vi "2L04_%-ds-Interv_centre_de_moy_de_lg_n_sigma.vi"(0 "xi":dbl[](array[numeric]), 1 "ni":i16[](array[numeric]), 2 "n":i16, 3 "Moyenne":dbl, 4 "Sigma":dbl) -> (7 "% de +/- n.sigma":dbl, 8 "i deb":i32, 9 "i fin":i32)   [LabVIEW 2010, in "lv_02.lvlib"]
doc: "Dans une distribution gaussienne LN(moyenne, sigma), on cherche dans une distribution expérimentale (xi,ni) le % de l'effectif dans un intervalle centré sur la moyenne à +/- n.sigma.\nSi la moyenne et sigma sont nuls alors, on calculera la moyenne et l'écart-type à partir de la distribution expérimentale."
uses:
  lv_02.lvlib
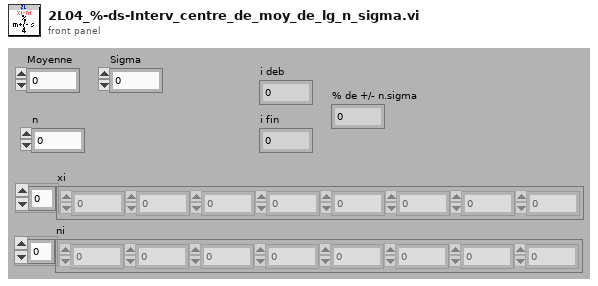
[diagram p1: front panel]
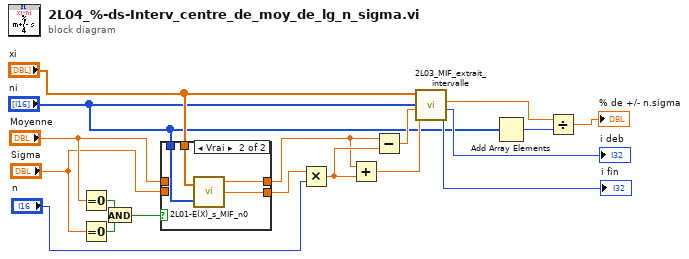
[diagram p0: block diagram]
diagram:
  n1 = Equal To 0?(x="Moyenne") -> (x = 0?=w9:bool)
  n2 = Equal To 0?(x="Sigma") -> (x = 0?=w8:bool)
  n3 = And(x=w9, y=w8) -> (x .and. y?=w7:bool)
  n4 = case shown="Vrai" w7 {
    tunnel: "xi" -> [_ w24]
    tunnel: "ni" -> [_ w23]
    tunnel: [w20 w22] -> w2
    tunnel: [w19 w21] -> w1
    tunnel: "Moyenne" -> [w20 _]
    tunnel: "Sigma" -> [w19 _]
    frame False {
    }
    frame True {
      n5 = call "2L01-E(X)_s_MIF_n0.vi"("ni"=w23, "xic"=w24) -> ("s"=w21:dbl, "E(X)"=w22:dbl)  [unwired: 1 out]
    }
  }
  n6 = Multiply(x=w1, y="n") -> (x*y=w18:dbl)
  n7 = Add(x=w2, y=w18) -> (x+y=w15:dbl)
  n8 = Subtract(x=w2, y=w18) -> (x-y=w16:dbl)
  n9 = call "2L03_MIF_extrait_intervalle.vi"("X fin"=w15, "X deb"=w16, "N"="ni", "X"="xi") -> ("i fin"=→"i fin":i32, "i deb"=→"i deb":i32, "Cumul"=w14:dbl)  [unwired: 2 in, 3 out]
  n10 = Add Array Elements(numeric array="ni") -> (sum=w12:i16)
  n11 = Divide(x=w14, y=w12) -> (x/y=→"% de +/- n.sigma":dbl)
